vi "test.vi"() -> ()   [LabVIEW 2023]
uses:
  Configurations/Pressure Control CFG/Red-y Pressure Control CFG.lvclass
  Configuration/Configuration JSON/Configuration JSON Base/CFG JSON.lvclass
  Configurations/Pressure Control CFG/Read Write PE Input.ctl
  <userlib>/_OpenG.lib/lvdata/lvdata.llb/Type Descriptor Enumeration__ogtk.ctl
  <userlib>/_OpenG.lib/lvdata/lvdata.llb/openg_variant.lvlib
panel:
  out "Output":variant
  in  "error in":errorcluster
  out "error out":errorcluster
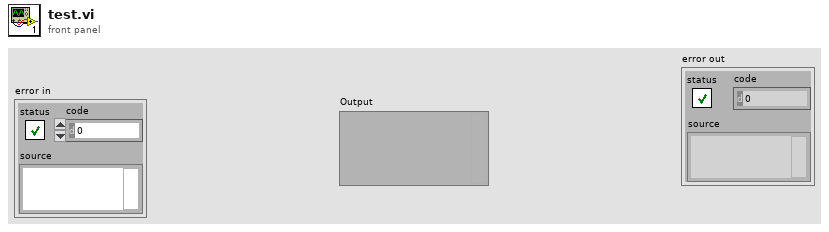
[diagram p1: front panel]
types:
  T1 = typedef "Read Write PE Input.ctl" = cluster{"Action":enum16{"Write", "Read"}, "Register":u16, "Type":T2, "Data":variant}
  T2 = typedef "openg_variant.lvlib/Type Descriptor Enumeration__ogtk.ctl" = enum8{"<Null>", "I8", "I16", "I32", "I64", "U8", "U16", "U32", "U64", "SGL", "DBL", "EXT", "CSG", "CDB", "CXT", "0x0F", "0x10", "0x11", "0x12", "0x13", "0x14", "Enum U8", "Enum U16", "Enum U32", "Enum U64", "SGL PQ", "DBL PQ", "EXT PQ", "CSG PQ", "CDB PQ", "CXT PQ", "0x1F", "0x20", "Boolean", "0x22", "0x23", "0x24", "0x25", "0x26", "0x27", "0x28", "0x29", "0x2A", "0x2B", "0x2C", "0x2D", "0x2E", "0x2F", "String", "0x31", "Path", "Pict", "0x34", "0x35", "0x36", "DAQ", "0x38", "0x39", "0x3A", "0x3B", "0x3C", "0x3D", "0x3E", "0x3F", "Array", "0x41", "0x42", "0x43", "0x44", "0x45", "0x46", "0x47", "0x48", "0x49", "0x4A", "0x4B", "0x4C", "0x4D", "0x4E", "0x4F", "Cluster", "0x51", "0x52", "Variant", "Waveform", "0x55", "0x56", "0x57", "0x58", "0x59", "0x5A", "0x5B", "0x5C", "0x5D", "0x5E", "Fixed Point", "0x60", "0x61", "0x62", "0x63", "0x64", "0x65", "0x66", "0x67", "0x68", "0x69", "0x6A", "0x6B", "0x6C", "0x6D", "0x6E", "0x6F", "Refnum", "0x71", "0x72", "Set Collection", "Map Collection"}
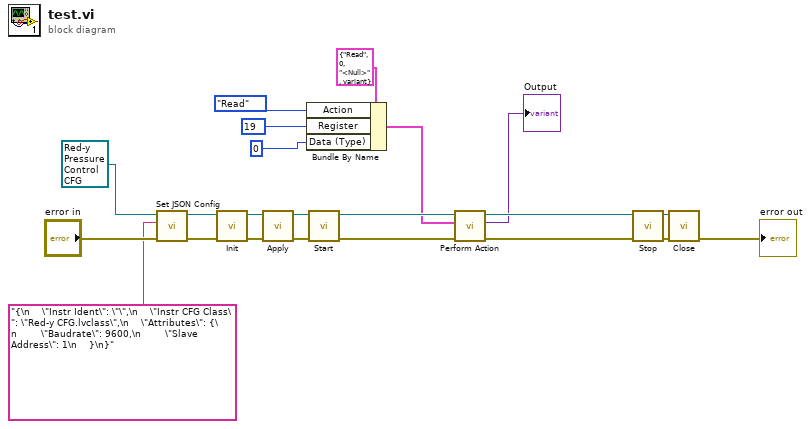
[diagram p0: block diagram]
diagram:
  n1 = call "Set JSON Config.vi"("error in (no error)"="error in", "<JSON>Config>"="{\n    \"Instr Ident\": \"\",\n    \"Instr CFG Class\": \"Red-y CFG.lvclass\",\n    \"Attributes\": {\n        \"Baudrate\": 9600,\n        \"Slave Address\": 1\n    }\n}", "CFG Base in"=refnum<class "Red-y Pressure Control CFG.lvclass"> refnum) -> ("error out"=w20:errorcluster, "CFG Base out"=w18:refnum<class "Red-y Pressure Control CFG.lvclass">)  [unwired: 7 in]
  n2 = call-dynamic "Init.vi"("error in"=w20, "CFG Base in"=w18) -> ("error out"=w22:errorcluster, "CFG Base out"=w3:refnum<class "Red-y Pressure Control CFG.lvclass">)  [unwired: 8 in]
  n3 = call-dynamic "Apply.vi"("error in"=w22, "Red-y Read Write CFG in"=w3) -> ("error out"=w4:errorcluster, "Red-y Read Write CFG out"=w2:refnum<class "Red-y Pressure Control CFG.lvclass">)  [unwired: 8 in]
  n4 = Bundle By Name(cluster=T1 {"Action"=enum."Read", "Register"=0, "Type"=enum."<Null>", "Data"=variant}, "Action"=enum16{"Write", "Read"}."Read", "Register"=u16 19 ("Register Start Address"), "Data (Type)"=u16 0) -> (w6:T1)
  n5 = call-dynamic "Start.vi"("error in"=w4, "Red-y Read Write CFG in"=w2) -> ("error out"=w15:errorcluster, "Red-y Read Write CFG out"=w11:refnum<class "Red-y Pressure Control CFG.lvclass">)  [unwired: 8 in]
  n6 = call-dynamic "Perform Action.vi"("error in"=w15, "Input"=w6, "Red-y Read Write CFG in"=w11) -> ("error out"=w12:errorcluster, "Output"=→"Output":variant, "Red-y Read Write CFG out"=w10:refnum<class "Red-y Pressure Control CFG.lvclass">)  [unwired: 6 in]
  n7 = call-dynamic "Stop.vi"("error in"=w12, "Red-y Read Write CFG in"=w10) -> ("error out"=w14:errorcluster, "Red-y Read Write CFG out"=w13:refnum<class "Red-y Pressure Control CFG.lvclass">)  [unwired: 8 in]
  n8 = call-dynamic "Close.vi"("error in"=w14, "Red-y Read Write CFG in"=w13) -> ("error out"=→"error out":errorcluster)  [unwired: 8 in, 1 out]
